vi "getUnrestrictedChannelArray.vi"(8 "error in (no error)":errorcluster, 11 "deviceDataBase in":refnum<class "deviceDataBase.lvclass">) -> (0 "error out":errorcluster, 2 "ChannelArray.lvclass":refnum<class "ChannelArray.lvclass">, 3 "deviceDataBase out":refnum<class "deviceDataBase.lvclass">)   [LabVIEW 2011, in "Tools.lvlib" / "DatabaseHelpers.lvlib" / "deviceDataBase.lvclass"]
doc: "Gets the unrestricted Channels from database"
uses:
  deviceDataBase.lvclass
  Database Objects/ChannelArray/ChannelArray.lvclass
  deviceDataBase.lvclass/deviceDataBase.ctl
  Database Objects/DeviceArray/DeviceArray.lvclass
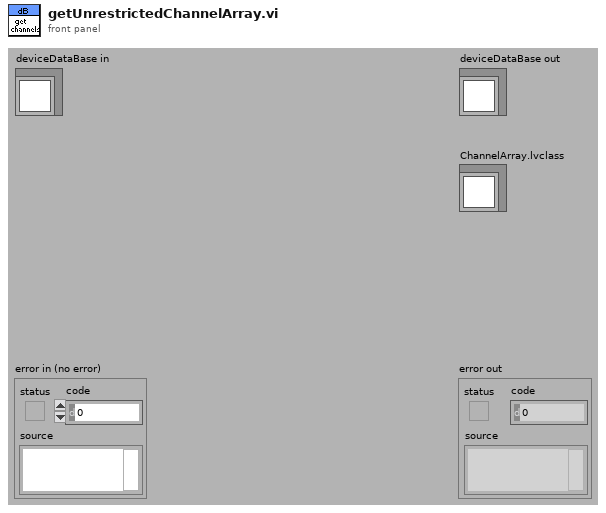
[diagram p1: front panel]
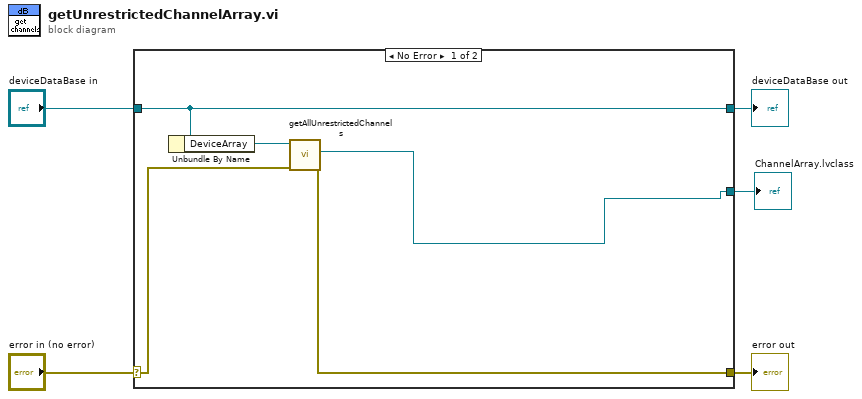
[diagram p0: block diagram]
diagram:
  n1 = case shown="No Error" "error in (no error)" {
    selector: "error in (no error)" -> [w8 w12]
    tunnel: [w7 w12] -> w4
    tunnel: [w10 w11] -> w2
    tunnel: "deviceDataBase in" -> [w10 w11]
    tunnel: [w6 _] -> w1
    frame No Error {
      n2 = Unbundle By Name(w10) -> ("DeviceArray"=w9:refnum<class "DeviceArray.lvclass">)
      n3 = call "getAllUnrestrictedChannels.vi"("error in (no error)"=w8, "DeviceArray in"=w9) -> ("error out"=w7:errorcluster, "ChannelArray.lvclass"=w6:refnum<class "ChannelArray.lvclass">)  [unwired: 7 in, 1 out]
    }
    frame Error {
    }
  }
  "error out" <- w4
  "deviceDataBase out" <- w2
  "ChannelArray.lvclass" <- w1
